vi "ConcatPaths.vi"(1 "Path2":string, 2 "Path1":string) -> (0 "Path1/Path2":string)   [LabVIEW 2017]
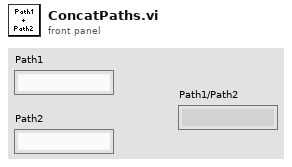
[diagram p1: front panel]
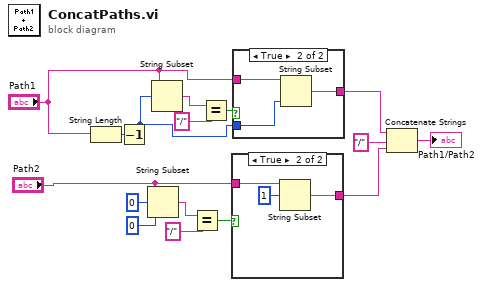
[diagram p0: block diagram]
diagram:
  n1 = String Length(string="Path1") -> (length=w16:i32)
  n2 = Decrement(x=w16) -> (x-1=w5:i32)
  n3 = String Subset(string="Path2", offset (0)=0, length (rest)=0 ("length (rest)")) -> (substring=w10:string)
  n4 = String Subset(string="Path1", offset (0)=w5) -> (substring=w15:string)  [unwired: 1 in]
  n5 = Equal?(x=w10, y="/") -> (x = y?=w8:bool)
  n6 = Equal?(x=w15, y="/") -> (x = y?=w7:bool)
  n7 = case shown="True" w8 {
    tunnel: "Path2" -> [w17 w20]
    tunnel: [w17 w18] -> w2
    frame False {
    }
    frame True {
      n8 = String Subset(string=w20, offset (0)=1) -> (substring=w18:string)  [unwired: 1 in]
    }
  }
  n9 = case shown="True" w7 {
    tunnel: "Path1" -> [w21 w24]
    tunnel: [w21 w23] -> w3
    tunnel: w5 -> [_ w22]
    frame False {
    }
    frame True {
      n10 = String Subset(string=w24, length (rest)=w22) -> (substring=w23:string)  [unwired: 1 in]
    }
  }
  n11 = Concatenate Strings(w3, "/" ("f"), w2) -> (→"Path1/Path2":string)
